vi "clientstreaming_client.vi"() -> ()   [LabVIEW 2019]
uses:
  Generated_client/RPC Messages/routeguide_Color.ctl
  Generated_client/RPC Messages/routeguide_request.ctl
  Generated_client/Generated_client.lvlib
panel:
  out "response_color":T1
  out "response_message":string
  out "response_number":i32
  out "error out":errorcluster
  in  "num_requests":i32
  in  "request_color":T1
  in  "request_message":string
  in  "request_number":i32
  in  "error in":errorcluster
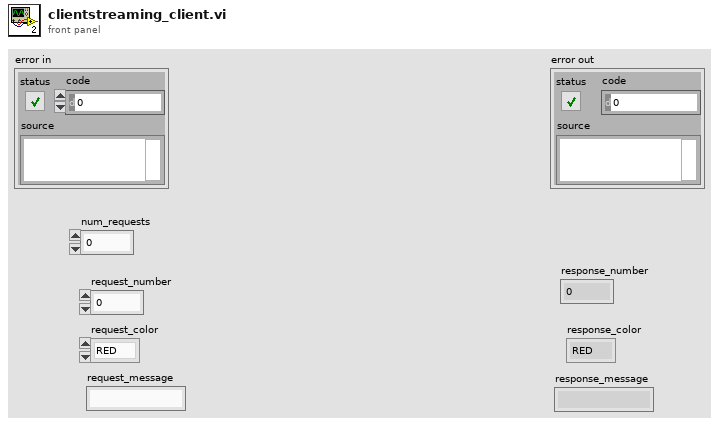
[diagram p1: front panel]
types:
  T1 = typedef "Generated_client.lvlib/routeguide_Color.ctl" = enum32{"RED", "GREEN", "BLUE"}
  T2 = typedef "grpc-lvsupport-release.lvlib/grpcId.ctl" = u64
  T3 = typedef "Generated_client.lvlib/routeguide_request.ctl" = cluster{"request_number":i32, "request_message":string, "request_color":T1}
  T4 = typedef "Generated_client.lvlib/routeguide_response.ctl" = cluster{"response_number":i32, "response_message":string, "response_color":T1}
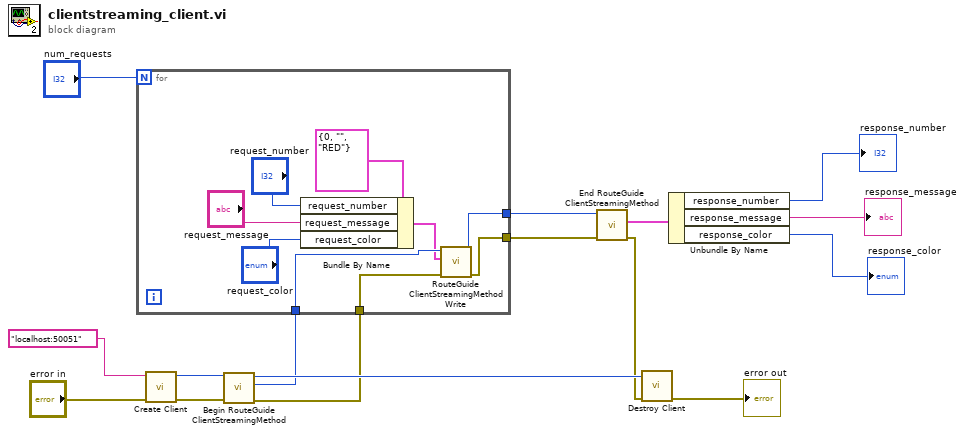
[diagram p0: block diagram]
diagram:
  n1 = call "Create Client.vi"("error in"="error in", "address"="localhost:50051") -> ("error out"=w14:errorcluster, "gRPC ID Out"=w15:T2)  [unwired: 8 in]
  n2 = call "Begin RouteGuide ClientStreamingMethod.vi"("error in"=w14, "gRPC ID"=w15) -> ("error out"=w10:errorcluster, "Call Id Out"=w9:T2, "gRPC ID out"=w13:T2)  [unwired: 7 in]
  n3 = for {
    N: "num_requests" -> [_]
    tunnel: w10 -> [w21]
    tunnel: w9 -> [w20]
    tunnel: [w19] -> w8
    tunnel: [w18] -> w7
    n4 = Bundle By Name(cluster=T3 {"request_number"=0, "request_message"="", "request_color"=enum."RED"} ("routeguide_request"), "request_number"="request_number", "request_message"="request_message", "request_color"="request_color") -> (w17:T3)
    n5 = call "RouteGuide ClientStreamingMethod Write.vi"("error in"=w21, "Request Data"=w17, "Call ID in"=w20) -> ("error out"=w19:errorcluster, "Call ID"=w18:T2)  [unwired: 6 in, 1 out]
  }
  n6 = call "End RouteGuide ClientStreamingMethod.vi"("error in"=w8, "Call ID in"=w7) -> ("error out"=w11:errorcluster, "Response Data"=w2:T4)  [unwired: 7 in, 1 out]
  n7 = call "Destroy Client.vi"("error in"=w11, "gRPC ID"=w13) -> ("error out"=→"error out":errorcluster)  [unwired: 9 in]
  n8 = Unbundle By Name(w2) -> ("response_number"=→"response_number":i32, "response_message"=→"response_message":string, "response_color"=→"response_color":T1)
